vi "DC Attenuation Flatten Test Parameters.vi"(7 "Test Configuration (\"\")":string, 9 "error in (no error)":errorcluster, 10 "Parameter Variant":variant) -> (1 "error out":errorcluster, 2 "Parameter String":string)   [LabVIEW 2011]
uses:
  TypeDefs/DCA Test Parameters.ctl
  TypeDefs/DCA Stimulus Parameters.ctl
  TypeDefs/DCA Measurement Cluster.ctl
  TypeDefs/DCA Topology.ctl
  TypeDefs/DCA Attenuation Calculation.ctl
  TypeDefs/DCA Limit.ctl
  TypeDefs/DCA Limit Quantity.ctl
  TypeDefs/DCA Limit Comparison.ctl
  TypeDefs/DCA Limit Operation.ctl
  Test Referential Limit.ctl
  TypeDefs/DCA Calibration State.ctl
  DC Attenuation Version.vi
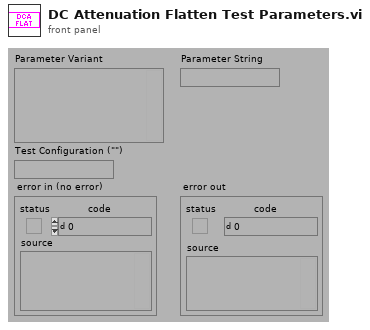
[diagram p1: front panel]
types:
  T1 = typedef "DCA Test Parameters.ctl" = cluster{"Stimulus":T2, "Measurement":T3, "Limits":T6[], "Normalization":T11}
  T2 = typedef "DCA Stimulus Parameters.ctl" = cluster{"Use Instrument":bool, "Normalize":bool, "Blank Screen":bool, "Measurement Type":enum16{"Voltage DC", "Voltage DC Ratio", "Voltage AC", "Current DC", "Current AC", "Resistance", "Fresistance", "Frequency", "Period", "Continuity", "Diode"}, "Range":enum16{"Auto", "Minimum", "Maximum", "100", "1,000", "10,000", "100,000", "1,000,000", "10,000,000", "100,000,000"}, "Resolution":enum16{"Auto", "4 1/2", "5 1/2", "6 1/2"}}
  T3 = typedef "DCA Measurement Cluster.ctl" = cluster{"Topology":T4, "Lock Topology":bool, "ATTN Calc":T5, "Zo":dbl}
  T4 = typedef "DCA Topology.ctl" = enum32{"PI-Network", "T-Network"}
  T5 = typedef "DCA Attenuation Calculation.ctl" = enum32{"Power", "Voltage"}
  T6 = typedef "DCA Limit.ctl" = cluster{"Parameter":T7, "Comparison":T8, "Operation":T9, "Value":dbl, "Referential Limit":T10}
  T7 = typedef "DCA Limit Quantity.ctl" = enum16{"Attenuation", "Zin", "Zout", "R1", "R2", "R3", "Rab", "Rac", "Rbc"}
  T8 = typedef "DCA Limit Comparison.ctl" = enum16{">", ">=", "<", "<="}
  T9 = typedef "DCA Limit Operation.ctl" = enum16{"+", "-"}
  T10 = typedef "Test Referential Limit.ctl" = cluster{"Ref Limit":bool, "Ref Type":enum16{"Current", "Specify"}, "Model":string, "Serial":string, "Run Type":enum16{"Most Recent", "Run #", "Match Field"}, "Run":i32, "Field":string, "Field Value":string}
  T11 = typedef "DCA Calibration State.ctl" = cluster{"Normalized?":bool, "Rab Value":dbl, "Rac Value":dbl, "Rbc Value":dbl}
  T12 = typedef "OGAB Version.ctl" = cluster{"Version":string, "Build Number":u32, "Build Date/Time":dbl}
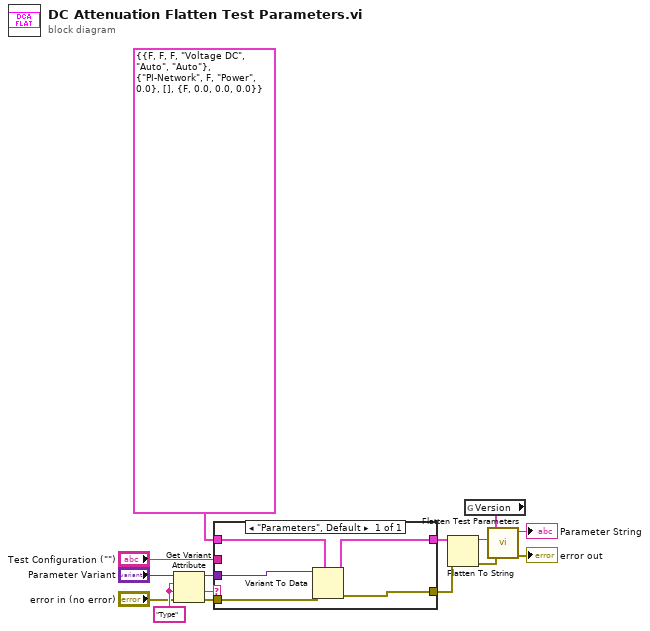
[diagram p0: block diagram]
diagram:
  w14 = "Type" ("name")
  n1 = Get Variant Attribute(Variant="Parameter Variant", name=w14, default value (empty Variant)=w14, error in="error in (no error)") -> (duplicate Variant=w3:variant, value=w2:string, error out=w7:errorcluster)  [unwired: 1 out]
  n2 = case shown="\"Parameters\", Default" w2 {
    tunnel: w3 -> [w20]
    tunnel: T1 {"Stimulus"={"Use Instrument"=FALSE, "Normalize"=FALSE, "Blank Screen"=FALSE, "Measurement Type"=enum."Voltage DC", "Range"=enum."Auto", "Resolution"=enum."Auto"}, "Measurement"={"Topology"=enum."PI-Network", "Lock Topology"=FALSE, "ATTN Calc"=enum."Power", "Zo"=0.0}, "Limits"=[], "Normalization"={"Normalized?"=FALSE, "Rab Value"=0.0, "Rac Value"=0.0, "Rbc Value"=0.0}} ("DCA Test Parameters") -> [w16]
    tunnel: [w17] -> w1
    tunnel: [w19] -> w4
    tunnel: w7 -> [w18]
    tunnel: "Test Configuration (\"\")" -> [_]
    frame "Parameters", Default {
      n3 = Variant To Data(error in=w18, type=w16, Variant=w20) -> (data=w17:T1, error out=w19:errorcluster)
    }
  }
  n4 = Flatten To String(anything=w1, error in (no error)=w4) -> (data string=w13:string, error out=w11:errorcluster)  [unwired: 3 out]
  n5 = global read "DC Attenuation Version.vi" "Version"() -> (w12:T12)
  n6 = call "Flatten Test Parameters.vi"("error in (no error)"=w11, "Flattened Test Parameters (\"\")"=w13, "Test Version"=w12) -> ("error out"=→"error out":errorcluster, "Flattened Test Parameters with Version"=→"Parameter String":string)  [unwired: 3 out]
